vi "FringeTracker-GetInfo.vi"(9 "error in (no error)":errorcluster) -> (2 "FringeTrackerInfo":T1={"Readout"={"Readout"=100, "Deglitch"=10, "Framerate"=200.0, "Bank"=2}, "OPD stroke"=0.0, "OPD per pixel"=0.0}, 6 "error out":errorcluster)   [LabVIEW 2009]
uses:
  Controls/FringeTrackerInfo.ctl
  Nicmos/Controls/NICMOS.READOUT.ctl
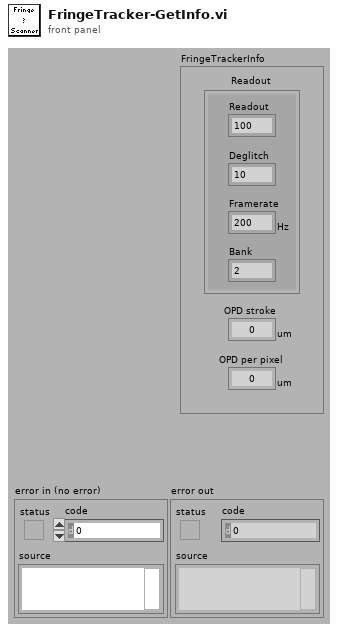
[diagram p1: front panel]
types:
  T1 = typedef "FringeTrackerInfo.ctl" = cluster{"Readout":T2, "OPD stroke":dbl[unit], "OPD per pixel":dbl[unit]}
  T2 = typedef "NICMOS.READOUT.ctl" = cluster{"Readout":i32, "Deglitch":i32, "Framerate":dbl[unit], "Bank":i32}
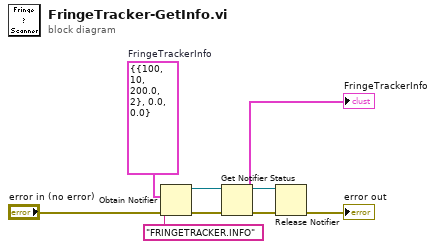
[diagram p0: block diagram]
diagram:
  w8 = T1 {"Readout"={"Readout"=100, "Deglitch"=10, "Framerate"=200.0, "Bank"=2}, "OPD stroke"=0.0, "OPD per pixel"=0.0}  # FringeTrackerInfo
  n1 = Obtain Notifier(name (unnamed)="FRINGETRACKER.INFO", notification data type=w8, error in (no error)="error in (no error)") -> (notifier out=w4:refnum<notifier>, error out=w3:errorcluster)  [unwired: 1 in, 1 out]
  n2 = Get Notifier Status(notifier=w4, error in (no error)=w3) -> (notifier out=w6:refnum<notifier>, current notification=→"FringeTrackerInfo":T1, error out=w7:errorcluster)  [unwired: 2 out]
  n3 = Release Notifier(notifier=w6, error in (no error)=w7) -> (error out=→"error out":errorcluster)  [unwired: 1 in, 2 out]
